vi "easySAM Load_Data2.vi"(9 "Load Data":bool=TRUE, 10 "Data References":T2, 11 "Data Parameters 0":T1) -> ()   [LabVIEW 2022 SP3]
uses:
  Data Record.ctl
  RF Data Value Reference.ctl
panel:
  in  "Save?":bool
  out "Samples":i32
  out "Number Pixel Y":i32
  out "Number Pixel X":i32
  out "All A-Scans":sgl[][](graph)
  out "File":path
  out "Data Parameters":T1
  # "easySAM Data Loading Module"
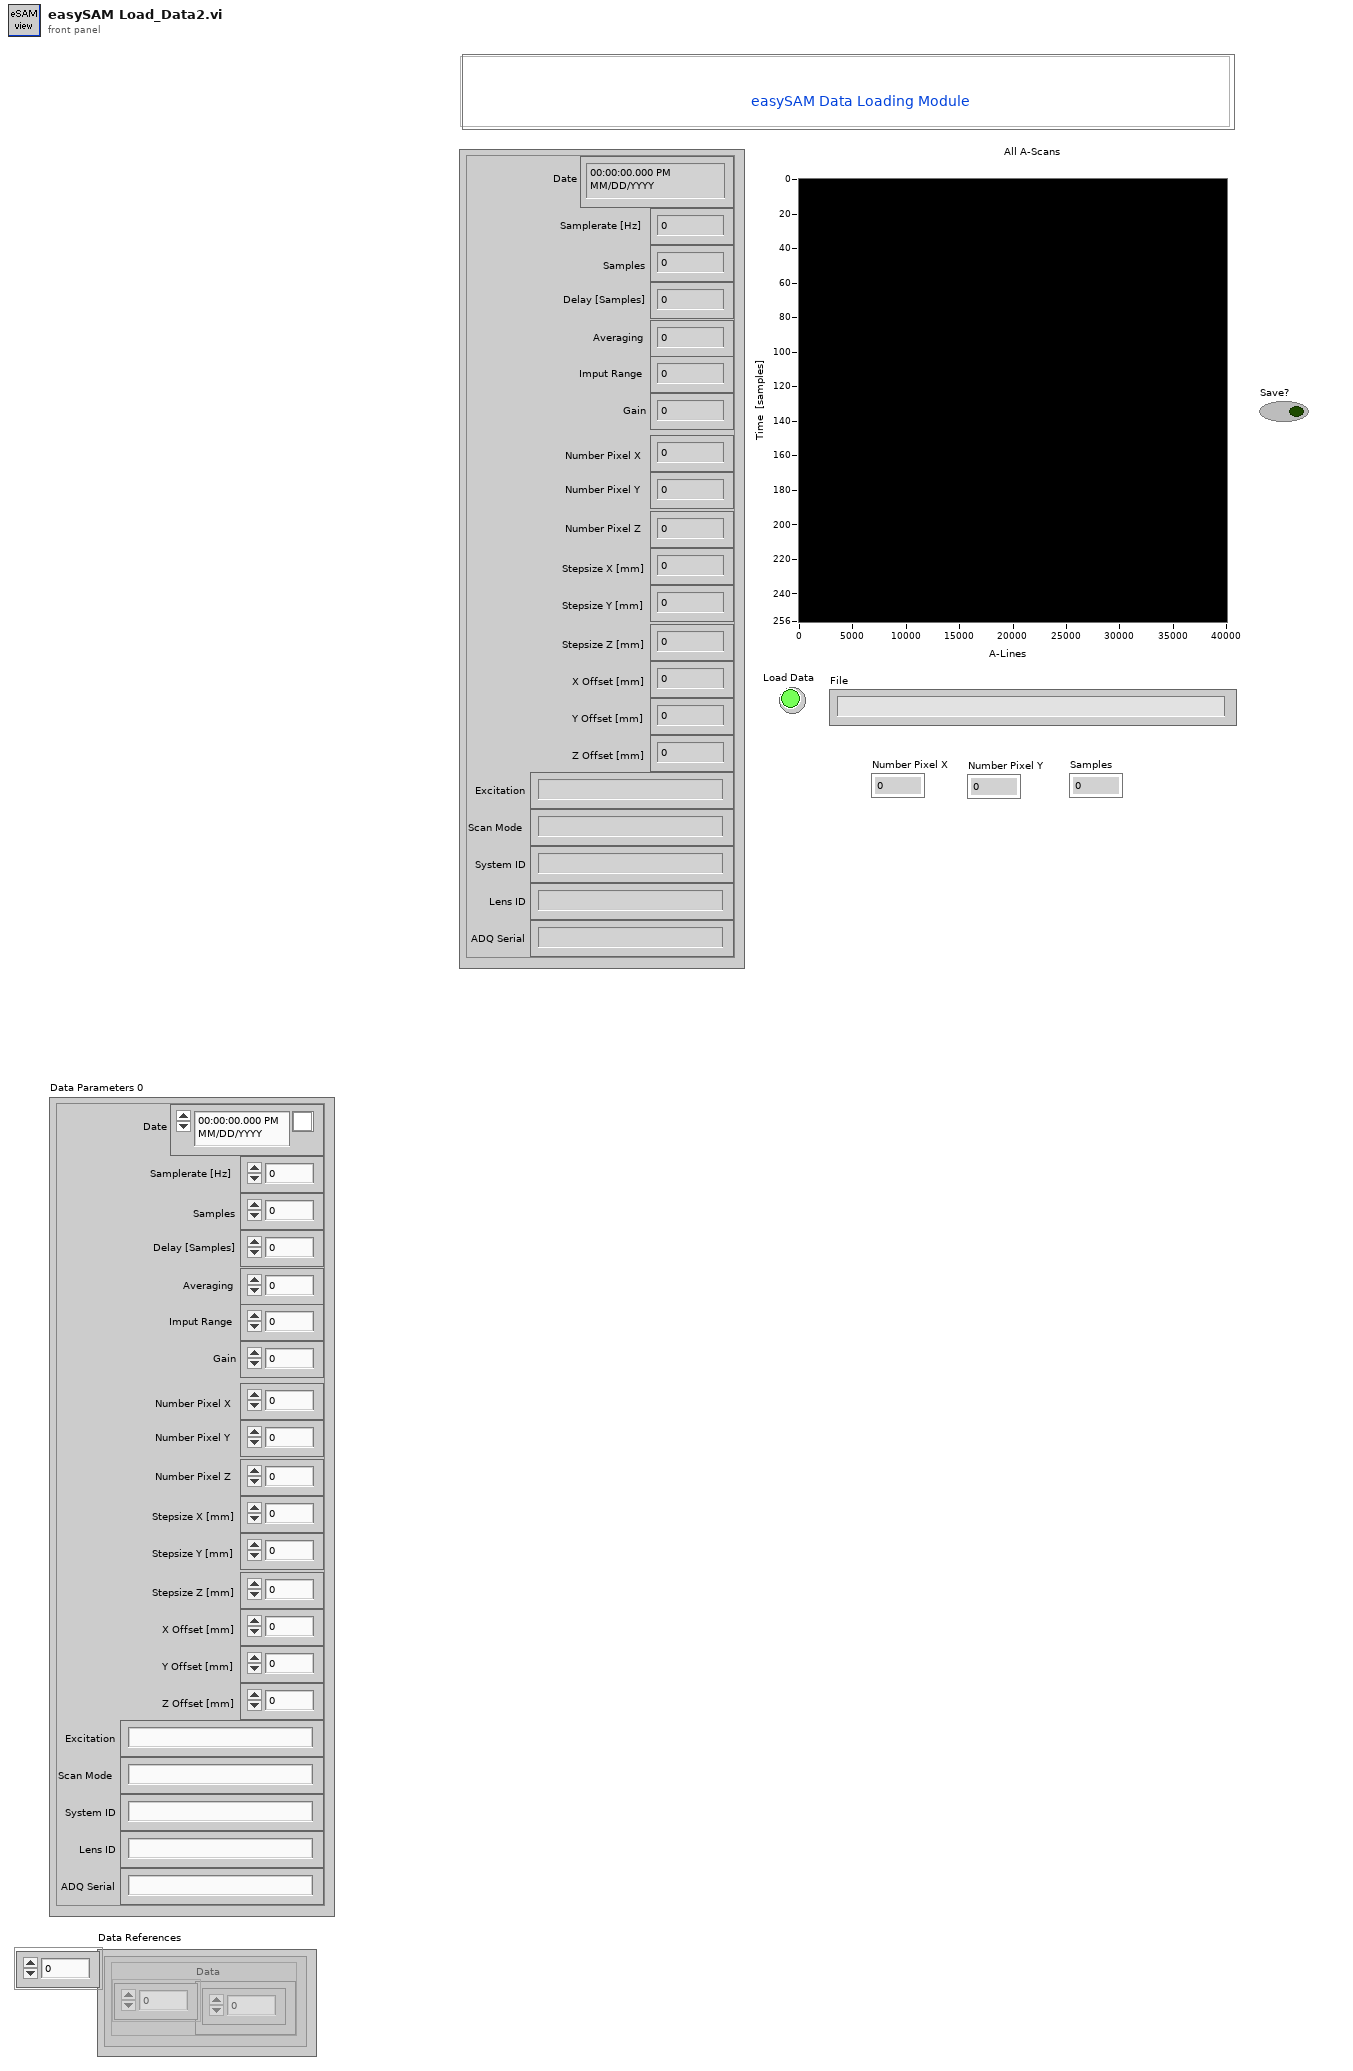
[diagram p1: front panel]
types:
  T1 = typedef "Data Record.ctl" = cluster{"Samplerate [Hz] ":dbl, "Delay [Samples]":i32, "Stepsize X [mm]":dbl, "Stepsize Y [mm]":dbl, "Z Offset [mm]":dbl, "Number Pixel X":i32, "Samples":i32, "Number Pixel Y":i32, "System ID":string, "Lens ID":string, "Date":timestamp, "X Offset [mm]":dbl, "Y Offset [mm]":dbl, "Scan Mode":string, "Excitation":string, "Gain":dbl, "Imput Range":dbl, "Averaging":i32, "ADQ Serial":string, "Stepsize Z [mm]":dbl, "Number Pixel Z":i32}
  T2 = typedef "RF Data Value Reference.ctl" = cluster{"Data":sgl[]}[]
  T3 = enum16{"big-endian, network order", "native, host order", "little-endian"}
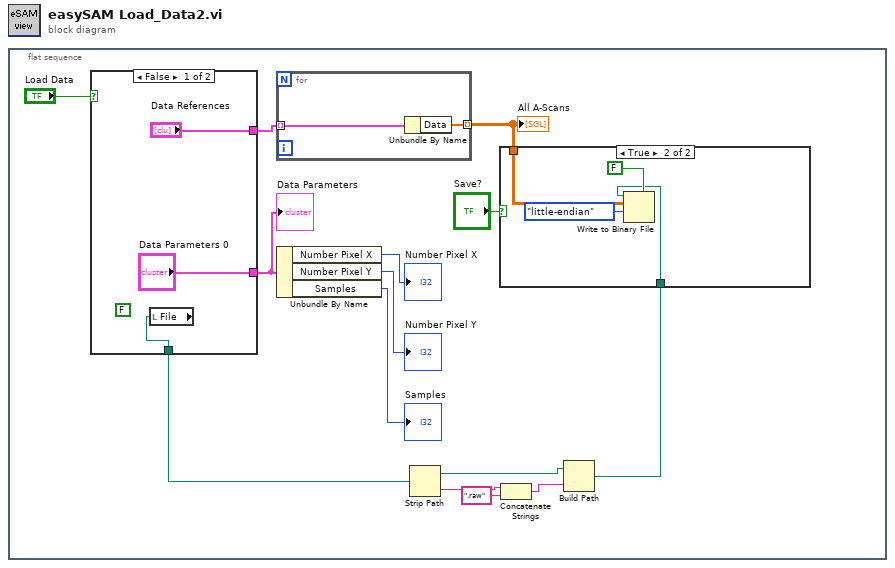
[diagram p0: block diagram]
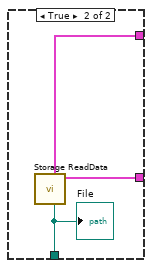
[diagram p3: hidden frame]
diagram:
  n1 = flat-sequence {
    frame #0 {
      n2 = case shown="False" "Load Data" {
        tunnel: ["Data Parameters 0" w23] -> w14
        tunnel: ["Data References" w24] -> w13
        tunnel: [w19 w22] -> w7
        frame False {
          (unwired) FALSE ("cancelled")
          n3 = local read "File"() -> (w19:path)
        }
        frame True {
          n4 = call "Storage ReadData.vi"() -> ("Acoustic Data"=w23:T1, "path"=w22:path, "Data Referenzen"=w24:T2)  [unwired: 6 in, 3 out]
          "File" <- w22
        }
      }
      "Data Parameters" <- w14
      n5 = for {
        tunnel: w13 -> [w26] mode=indexing
        tunnel: [w25] -> w8 mode=indexing
        n6 = Unbundle By Name(w26) -> ("Data"=w25:sgl[])
      }
      "All A-Scans" <- w8
      n7 = Unbundle By Name(w14) -> ("Number Pixel X"=→"Number Pixel X":i32, "Number Pixel Y"=→"Number Pixel Y":i32, "Samples"=→"Samples":i32)
      n8 = Strip Path(path=w7) -> (stripped path=w3:path, name=w6:string)
      n9 = Concatenate Strings(w6, ".raw" ("string")) -> (w4:string)
      n10 = Build Path(base path=w3, name or relative path=w4) -> (appended path=w2:path)
      n11 = case shown="True" "Save?" {
        tunnel: w8 -> [_ w18]
        tunnel: w2 -> [_ w15]
        frame False {
        }
        frame True {
          n12 = Write to Binary File(file (use dialog)=w15, data=w18, 5:FALSE ("prepend array or string size? (T)"), 9:T3."little-endian" ("byte order (0:big-endian, network order)")) -> ()  [unwired: 2 in, 3 out]
        }
      }
    }
  }
